vi "Acquire and Log Data.vi"(7 "DAQmx Task Name":refnum<k21>, 8 "error in (no error)":errorcluster, 9 "Number of Blocks Saved in":i32, 10 "Acquisition and Logging Configuration":T1={"Data Rate (Hz)"=1.0, "Samples per Read"=0, "Number of Reads to Save"=0, "Data File Name"="", "TDMS Properties"=[], "Number of Channels"=4, "Channel Scale Array"=[0.0, 0.0, 0.0, 0.0], "Channel Names"=[], "Trigger - RMS Value"=0.0, "Trigger - Channel"=0, "Trigger - Time (Minute)"=0, "Enable RMS Trigger"=FALSE, "Enable Time Trigger"=FALSE, "Always Log"=FALSE}, 11 "TDMS File Reference":refnum<k34>) -> (0 "error out":errorcluster, 1 "Number of Blocks Saved out":i32, 3 "Logging Complete?":bool)   [LabVIEW 2022 SP3]
uses:
  controls/Acquisition and Logging Configuration.ctl
  controls/TDMS Properties.ctl
  <vilib>/Analysis/5stat.llb/RMS (DBL).vi
  Globals/Global - Monitoring Variables.vi
  <vilib>/Analysis/NI_AALPro.lvlib
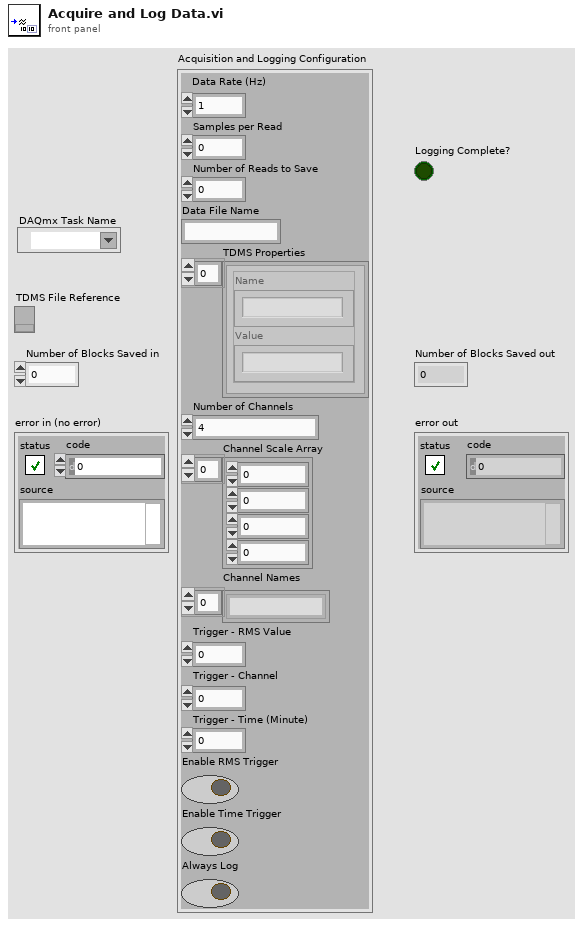
[diagram p1: front panel]
types:
  T1 = typedef "Acquisition and Logging Configuration.ctl" = cluster{"Data Rate (Hz)":dbl, "Samples per Read":i32, "Number of Reads to Save":i32, "Data File Name":string, "TDMS Properties":T2[], "Number of Channels":i32, "Channel Scale Array":dbl[], "Channel Names":string[], "Trigger - RMS Value":dbl, "Trigger - Channel":i32, "Trigger - Time (Minute)":i32, "Enable RMS Trigger":bool, "Enable Time Trigger":bool, "Always Log":bool}
  T2 = typedef "TDMS Properties.ctl" = cluster{"Name":string, "Value":string}
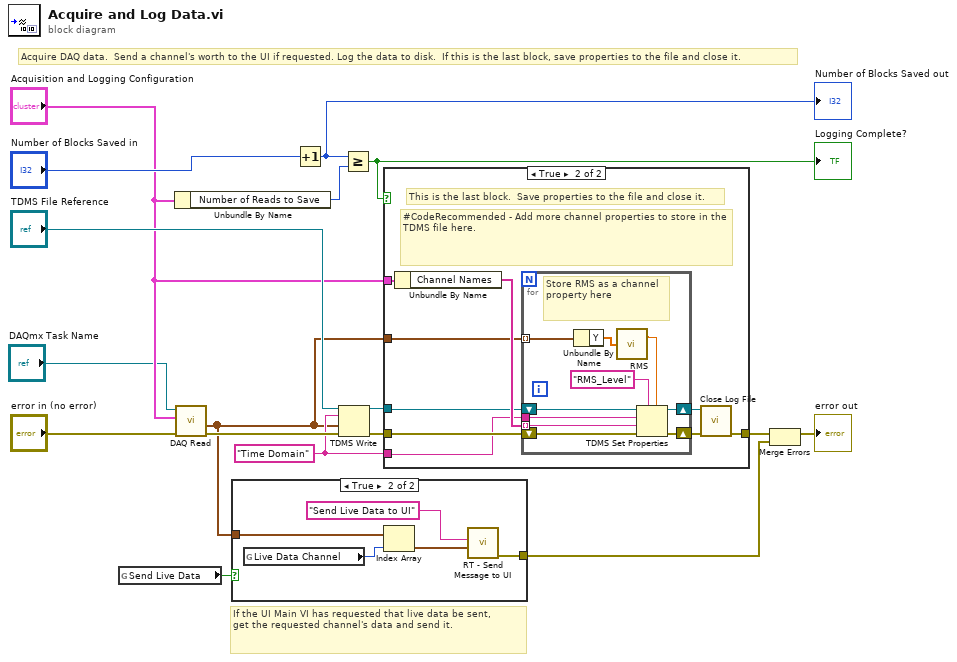
[diagram p0: block diagram]
diagram:
  w6 = "Time Domain" ("group name in (Untitled)")
  # "Acquire DAQ data.  Send a channel's worth to the UI if requested. Log the data to disk.  If this is the last block, save properties to the file and close it."
  # "If the UI Main VI has requested that live data be sent,\nget the requested channel's data and send it."
  n1 = global read "Global - Monitoring Variables.vi" "Send Live Data"() -> (w4:bool)
  n2 = Unbundle By Name("Acquisition and Logging Configuration") -> ("Number of Reads to Save"=w12:i32)
  n3 = call "DAQ Read.vi"("error in (no error)"="error in (no error)", "Acquisition and Logging Configuration"="Acquisition and Logging Configuration", "DAQmx Task Name"="DAQmx Task Name") -> ("error out"=w16:errorcluster, "Waveform Data"=w3:waveform(dbl)[])  [unwired: 6 in, 1 out]
  n4 = case shown="True" w4 {
    tunnel: w3 -> [_ w22]
    tunnel: [_ w19] -> w2
    frame False {
    }
    frame True {
      n5 = global read "Global - Monitoring Variables.vi" "Live Data Channel"() -> (w21:u32)
      n6 = Index Array(array=w22, index=w21) -> (element=w20:waveform(dbl))
      n7 = call "RT - Send Message to UI.vi"("Message Data"=w20, "Message"="Send Live Data to UI" ("group name in (Untitled)")) -> ("error out"=w19:errorcluster)  [unwired: 9 in]
    }
  }
  n8 = Increment(x="Number of Blocks Saved in") -> (x+1=w13:i32)
  "Number of Blocks Saved out" <- w13
  n9 = TDMS Write(0:"TDMS File Reference", 5:w6, 9:w3, 11:w16) -> (4:w10:refnum<k34>, 15:w9:errorcluster)  [unwired: 2 in, 2 out]
  n10 = Greater Or Equal?(x=w13, y=w12) -> (x >= y?=w11:bool)
  "Logging Complete?" <- w11
  n11 = case shown="True" w11 {
    tunnel: w10 -> [_ w28]
    tunnel: w9 -> [w23 w31]
    tunnel: [w23 w24] -> w8
    tunnel: "Acquisition and Logging Configuration" -> [_ w32]
    tunnel: w6 -> [_ w27]
    tunnel: w3 -> [_ w26]
    frame False {
      # "Do not finish the file.  This is not the last block."
    }
    frame True {
      # "This is the last block.  Save properties to the file and close it."
      # "#CodeRecommended - Add more channel properties to store in the TDMS file here."
      n12 = Unbundle By Name(w32) -> ("Channel Names"=w29:string[])
      n13 = for {
        tunnel: w27 -> [w39]
        shift-right: [w41] -> w30
        shift-left: w31 -> [w40]
        tunnel: w29 -> [w38] mode=indexing
        tunnel: w26 -> [w35] mode=indexing
        shift-right: [w36] -> w25
        shift-left: w28 -> [w42]
        # "Store RMS as a channel property here"
        n14 = Unbundle By Name(w35) -> ("Y"=w34:dbl[])
        n15 = call-poly <vilib>:"RMS.vi"("X"=w34) -> ("rms value"=w33:dbl)  [unwired: 1 out]
        n16 = TDMS Set Properties(5:w33, 7:"RMS_Level" ("property names"), 8:w40, 9:w38, 10:w39, 11:w42) -> (0:w41:errorcluster, 3:w36:refnum<k34>)  [unwired: 2 out]
      }
      n17 = call "Close Log File.vi"("error in (no error)"=w30, "Log File"=w25) -> ("error out"=w24:errorcluster)  [unwired: 9 in]
    }
  }
  n18 = Merge Errors(w8, w2) -> (→"error out":errorcluster)
